vi "IterateControls.vi"(0 "Controls[] In":refnum<vi>[](array[refnum]), 5 "ControlDoBase in":refnum<class "ControlActionBase.lvclass">, 7 "Control Path":string[](array[string]), 11 "error in (no error)":errorcluster) -> (4 "Controls[] Out":refnum<vi>[](array[refnum]), 6 "ControlDoBase out":refnum<class "ControlActionBase.lvclass">, 15 "error out":errorcluster)   [LabVIEW 2016, in "ControlActionBase.lvclass"]
doc: "This VI sets value for the controls present n other VI"
uses:
  ControlActionBase.lvclass
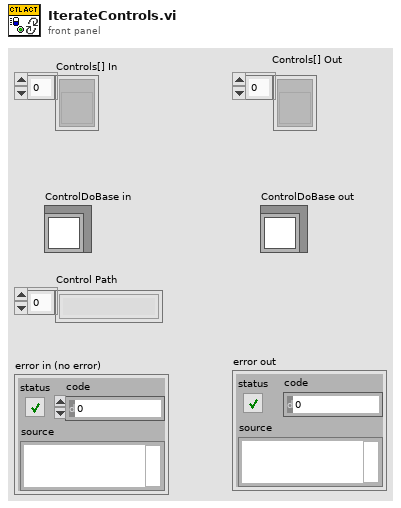
[diagram p1: front panel]
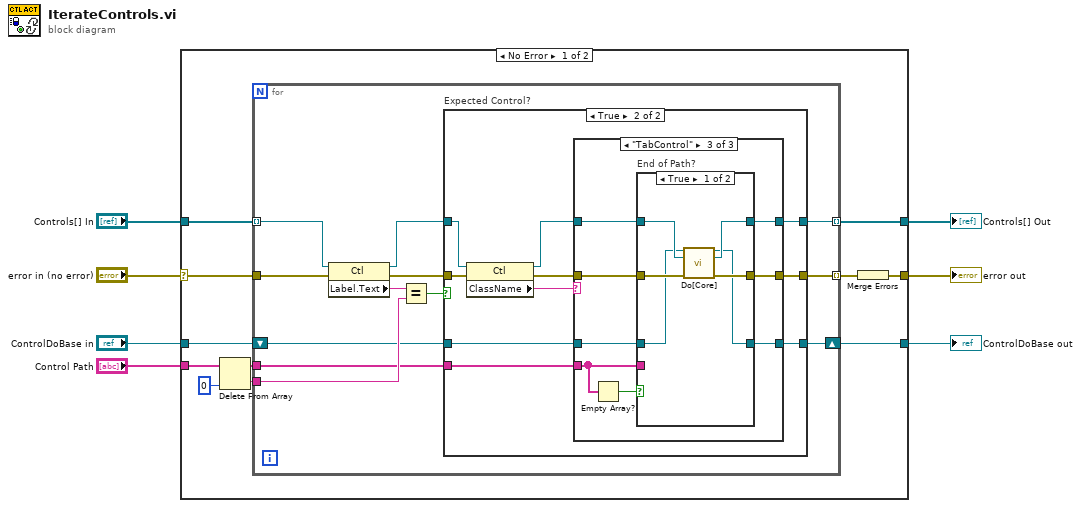
[diagram p0: block diagram]
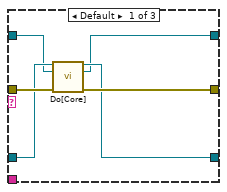
[diagram p3: hidden frame]
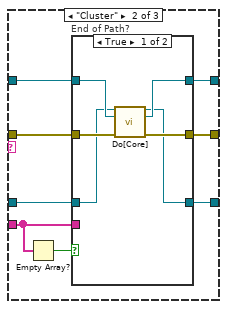
[diagram p4: hidden frame]
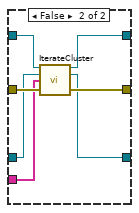
[diagram p5: hidden frame]
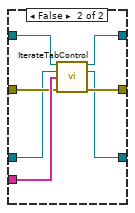
[diagram p6: hidden frame]
diagram:
  n1 = case shown="No Error" "error in (no error)" {
    selector: "error in (no error)" -> [w15 w93]
    tunnel: [w14 w93] -> w5
    tunnel: "Control Path" -> [w13 _]
    tunnel: "ControlDoBase in" -> [w17 w92]
    tunnel: "Controls[] In" -> [w9 w94]
    tunnel: [w8 w94] -> w2
    tunnel: [w18 w92] -> w1
    frame No Error {
      n2 = Delete From Array(array=w13, index=0) -> (deleted portion=w11:string, array with subset deleted=w12:string[])  [unwired: 1 in]
      n3 = for {
        shift-right: [w21] -> w18
        shift-left: w17 -> [w20]
        tunnel: w9 -> [w27] mode=indexing
        tunnel: [w23] -> w8 mode=indexing
        tunnel: [w30] -> w16 mode=indexing
        tunnel: w15 -> [w28]
        tunnel: w12 -> [w19]
        tunnel: w11 -> [w25]
        n4 = property class="Ctl"(reference=w27, error in=w28) -> (reference out=w24:refnum<vi>, error out=w26:errorcluster, "Label.Text"=w29:string)
        n5 = Equal?(x=w29, y=w25) -> (x = y?=w22:bool)
        n6 = case "Expected Control?" shown="True" w22 {
          tunnel: [w32 w43] -> w30
          tunnel: w26 -> [w32 w42]
          tunnel: w24 -> [w33 w40]
          tunnel: [w33 w38] -> w23
          tunnel: [w31 w35] -> w21
          tunnel: w20 -> [w31 w36]
          tunnel: w19 -> [_ w34]
          frame False {
          }
          frame True {
            n7 = property class="Ctl"(reference=w40, error in=w42) -> (reference out=w39:refnum<vi>, error out=w41:errorcluster, "ClassName"=w37:string)
            n8 = case shown="\"TabControl\"" w37 {
              tunnel: [w48 w54 w75] -> w43
              tunnel: w41 -> [w49 w57 w78]
              tunnel: w39 -> [w45 w56 w77]
              tunnel: [w44 w55 w76] -> w38
              tunnel: w36 -> [w47 w53 w74]
              tunnel: [w46 w52 w73] -> w35
              tunnel: w34 -> [_ w51 w72]
              frame Default {
                n9 = call-dynamic "Do[Core].vi"("ControlAction in"=w47, "Ctl Refnum in"=w45, "error in (no error)"=w49) -> ("ControlAction out"=w46:refnum<class "ControlActionBase.lvclass">, "Ctl Refnum out"=w44:refnum<vi>, "error out"=w48:errorcluster)  [unwired: 10 in]
              }
              frame "Cluster" {
                n10 = Empty Array?(array=w51) -> (empty?=w50:bool)
                n11 = case "End of Path?" shown="True" w50 {
                  tunnel: w57 -> [w63 w70]
                  tunnel: w56 -> [w60 w67]
                  tunnel: [w61 w66] -> w55
                  tunnel: [w62 w69] -> w54
                  tunnel: w53 -> [w59 w65]
                  tunnel: [w58 w64] -> w52
                  tunnel: w51 -> [_ w68]
                  frame True {
                    n12 = call-dynamic "Do[Core].vi"("ControlAction in"=w59, "Ctl Refnum in"=w60, "error in (no error)"=w63) -> ("ControlAction out"=w58:refnum<class "ControlActionBase.lvclass">, "Ctl Refnum out"=w61:refnum<vi>, "error out"=w62:errorcluster)  [unwired: 10 in]
                  }
                  frame False {
                    n13 = call "IterateCluster.vi"("Ctl Refnum in"=w67, "ControlDoBase in"=w65, "Control Path"=w68, "error in (no error)"=w70) -> ("Ctl Refnum out"=w66:refnum<vi>, "ControlDoBase out"=w64:refnum<class "ControlActionBase.lvclass">, "error out"=w69:errorcluster)  [unwired: 9 in]
                  }
                }
              }
              frame "TabControl" {
                n14 = Empty Array?(array=w72) -> (empty?=w71:bool)
                n15 = case "End of Path?" shown="True" w71 {
                  tunnel: w78 -> [w84 w90]
                  tunnel: w77 -> [w81 w85]
                  tunnel: [w82 w86] -> w76
                  tunnel: [w83 w89] -> w75
                  tunnel: w74 -> [w80 w88]
                  tunnel: [w79 w87] -> w73
                  tunnel: w72 -> [_ w91]
                  frame True {
                    n16 = call-dynamic "Do[Core].vi"("ControlAction in"=w80, "Ctl Refnum in"=w81, "error in (no error)"=w84) -> ("ControlAction out"=w79:refnum<class "ControlActionBase.lvclass">, "Ctl Refnum out"=w82:refnum<vi>, "error out"=w83:errorcluster)  [unwired: 10 in]
                  }
                  frame False {
                    n17 = call "IterateTabControl.vi"("Ctl Refnum in"=w85, "ControlDoBase in"=w88, "Control Path"=w91, "error in (no error)"=w90) -> ("Ctl Refnum out"=w86:refnum<vi>, "ControlDoBase out"=w87:refnum<class "ControlActionBase.lvclass">, "error out"=w89:errorcluster)  [unwired: 9 in]
                  }
                }
              }
            }
          }
        }
      }
      n18 = Merge Errors(w16) -> (w14:errorcluster)
    }
    frame Error {
    }
  }
  "error out" <- w5
  "Controls[] Out" <- w2
  "ControlDoBase out" <- w1
